vi "getObject.vi"(1 "lineStyle":T1 caption="stroke", 5 "error in (no error)":errorcluster) -> (14 "reference out":refnum<class "LineStyle.lvclass">, 19 "error out":errorcluster)   [LabVIEW 2016, in "LineStyle.lvclass"]
doc: "Gets an object"
uses:
  <resource>/Framework/Providers/Open_GDS/UML/LineStyle_class/LineStyle.lvclass
  <resource>/Framework/Providers/Open_GDS/UML/LineStyle_class/LineStyleType.ctl
  <resource>/Framework/Providers/Open_GDS/UML/LineStyle_class/LineStyle.lvclass/LineStyle.ctl
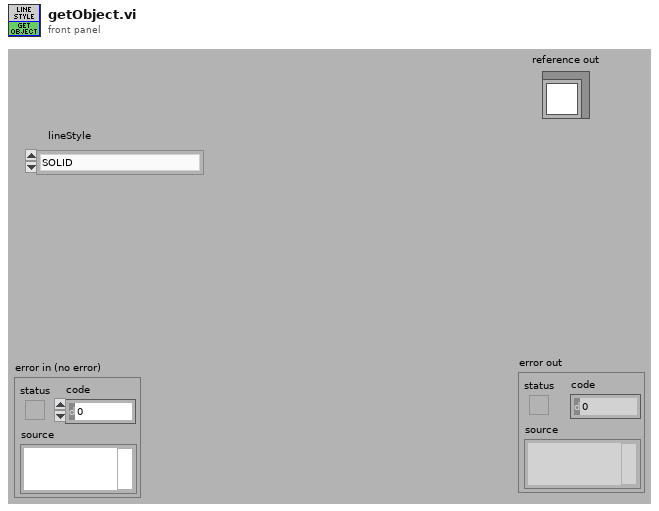
[diagram p1: front panel]
types:
  T1 = typedef "LineStyle.lvclass/LineStyleType.ctl" = enum16{"SOLID", "DOTTED"}
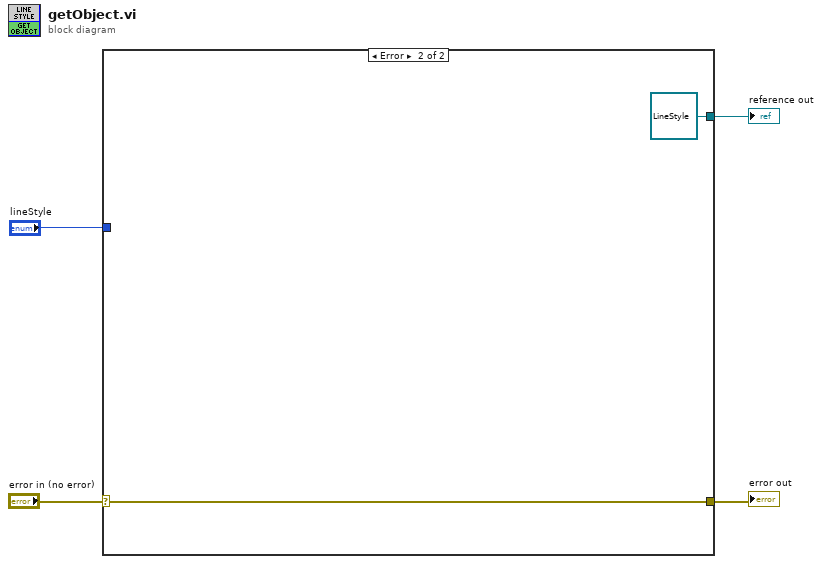
[diagram p0: block diagram]
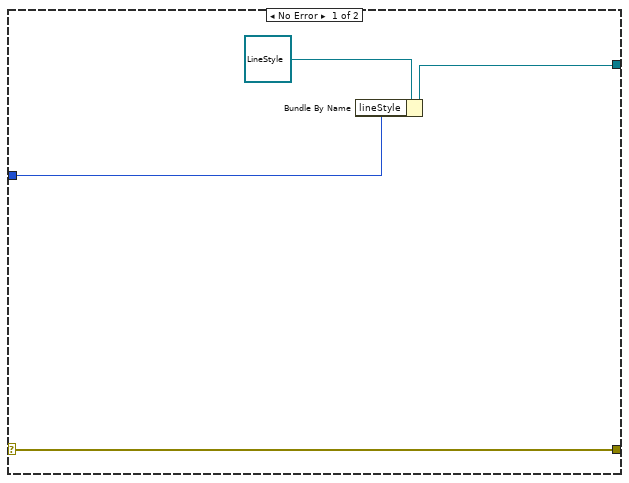
[diagram p2: hidden frame]
diagram:
  n1 = case shown="Error" "error in (no error)" {
    selector: "error in (no error)" -> [w5 w10]
    tunnel: [w5 w10] -> w3
    tunnel: [w6 refnum<class "LineStyle.lvclass"> refnum ("reference out")] -> w2
    tunnel: "lineStyle" -> [w7 _]
    frame No Error {
      n2 = Bundle By Name(cluster=refnum<class "LineStyle.lvclass"> refnum ("reference out"), "lineStyle"=w7) -> (w6:refnum<class "LineStyle.lvclass">)
    }
    frame Error {
    }
  }
  "reference out" <- w2
  "error out" <- w3
